vi "CorrectResponse.vi"(8 "error in (no error)":errorcluster, 11 "TrialBasedExperiment in":refnum<class "MatlabExperiment.lvclass">) -> (0 "error out":errorcluster, 3 "TrialBasedExperiment out":refnum<class "MatlabExperiment.lvclass">)   [LabVIEW 2010, in "MatlabExperiment.lvclass"]
uses:
  MatlabExperiment.lvclass
  TrialBasedExperimentObject/TrialBasedExperiment.lvclass
  Core SubVIs/Core SubVIs.lvlib
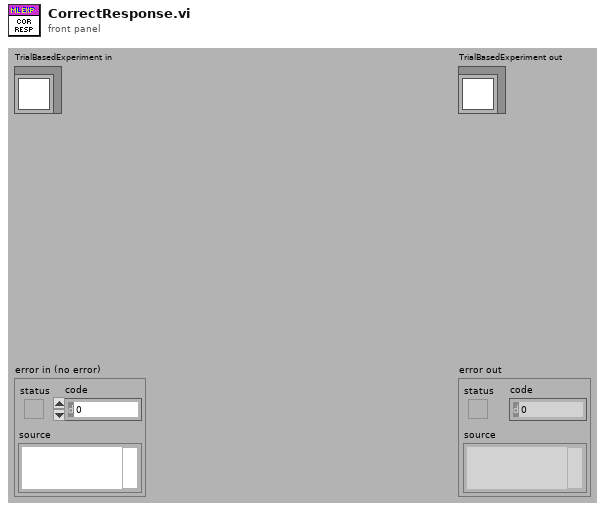
[diagram p1: front panel]
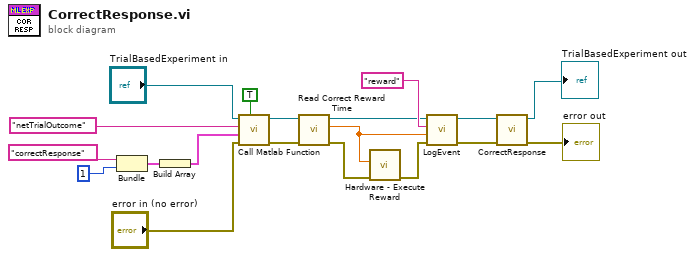
[diagram p0: block diagram]
diagram:
  n1 = Bundle("correctResponse", 1) -> (w14:cluster{string, i32})  [unwired: 1 out]
  n2 = Build Array(w14) -> (w13:cluster{string, i32}[])
  n3 = call-dynamic "Call Matlab Function.vi"("Timestamp"=TRUE, "error in (no error)"="error in (no error)", "Matlab Param Array"=w13, "Function name"="netTrialOutcome", "TrialBasedExperiment in"="TrialBasedExperiment in") -> ("error out"=w5:errorcluster, "TrialBasedExperiment out"=w2:refnum<class "MatlabExperiment.lvclass">)  [unwired: 3 in, 2 out]
  n4 = call-dynamic "Read Correct Reward Time.vi"("error in (no error)"=w5, "MatlabExperiment in"=w2) -> ("error out"=w4:errorcluster, "Correct Reward Time"=w3:dbl, "MatlabExperiment out"=w1:refnum<class "MatlabExperiment.lvclass">)  [unwired: 7 in]
  n5 = call "Hardware - Execute Reward.vi"("error in (no error)"=w4, "Reward Time (200 ms)"=w3) -> ("error out"=w11:errorcluster)  [unwired: 9 out]
  n6 = call-dynamic "LogEvent.vi"("error in (no error)"=w11, "eventInfo"=w3, "Event Name"="reward", "TrialBasedExperiment in"=w1) -> ("error out"=w10:errorcluster, "TrialBasedExperiment out"=w9:refnum<class "MatlabExperiment.lvclass">)  [unwired: 6 in]
  n7 = call-parent "CorrectResponse.vi"("error in (no error)"=w10, "TrialBasedExperiment in"=w9) -> ("error out"=→"error out":errorcluster, "TrialBasedExperiment out"=→"TrialBasedExperiment out":refnum<class "MatlabExperiment.lvclass">)  [unwired: 8 in]
